vi "Neilsetplot.vi"(6 "Set axes names":bool=TRUE, 7 "max # rows (-1:all)":i32=-1, 8 "error in":errorcluster, 9 "X-axis names":string[](array[string]), 10 "Plot names":string[](array[string]), 11 "XYGraph Refnum":refnum<vi>) -> (0 "error out":errorcluster, 3 "XYGraph Refnum out":refnum<vi>)   [LabVIEW 2015]
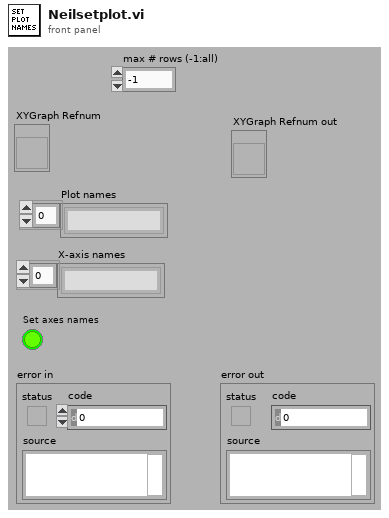
[diagram p1: front panel]
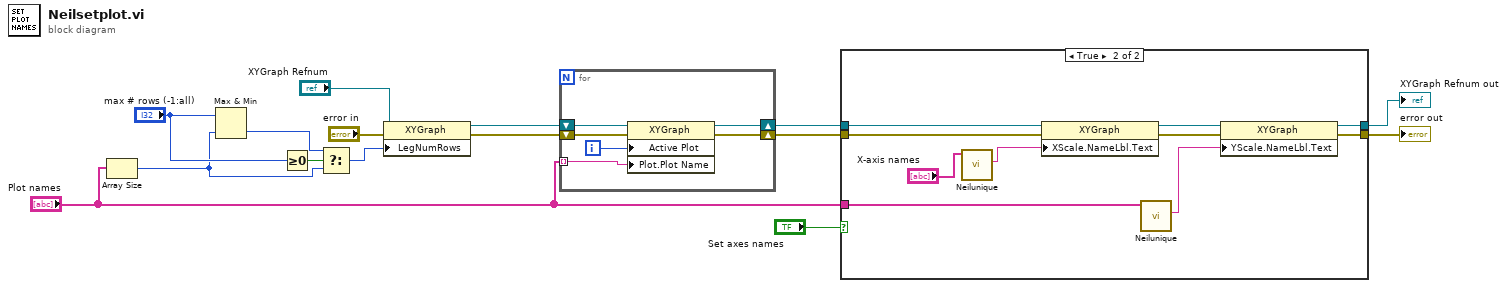
[diagram p0: block diagram]
diagram:
  n1 = Array Size(array="Plot names") -> (size(s)=w2:i32)
  n2 = Max & Min(x="max # rows (-1:all)", y=w2) -> (min(x,y)=w3:i32)  [unwired: 1 out]
  n3 = Greater Or Equal To 0?(x="max # rows (-1:all)") -> (x >= 0?=w4:bool)
  n4 = Select(t=w3, s=w4, f=w2) -> (s? t:f=w1:i32)
  n5 = property on="Property Node" class="XYGraph"(reference="XYGraph Refnum", error in="error in", "LegNumRows"=w1) -> (reference out=w11:refnum<vi>, error out=w15:errorcluster)
  n6 = for {
    shift-right: [w20] -> w13
    shift-left: w15 -> [w21]
    tunnel: "Plot names" -> [w18] mode=indexing
    shift-right: [w16] -> w10
    shift-left: w11 -> [w17]
    i -> [w19]
    n7 = property on="Property Node" class="XYGraph"(reference=w17, error in=w21, "Active Plot"=w19, "Plot.Plot Name"=w18) -> (reference out=w16:refnum<vi>, error out=w20:errorcluster)
  }
  n8 = case shown="True" "Set axes names" {
    tunnel: w13 -> [w23 w33]
    tunnel: w10 -> [w22 w32]
    tunnel: [w22 w29] -> w9
    tunnel: [w23 w28] -> w8
    tunnel: "Plot names" -> [_ w25]
    frame False {
    }
    frame True {
      n9 = call "Neilunique.vi"("Names"="X-axis names") -> ("Coma separated"=w26:string)  [unwired: 9 in, 1 out]
      n10 = property class="XYGraph"(reference=w32, error in=w33, "XScale.NameLbl.Text"=w26) -> (reference out=w30:refnum<vi>, error out=w31:errorcluster)
      n11 = call "Neilunique.vi"("Names"=w25) -> ("Coma separated"=w24:string)  [unwired: 9 in, 1 out]
      n12 = property class="XYGraph"(reference=w30, error in=w31, "YScale.NameLbl.Text"=w24) -> (reference out=w29:refnum<vi>, error out=w28:errorcluster)
    }
  }
  "error out" <- w8
  "XYGraph Refnum out" <- w9
